vi "ProgG_011_MG.vi"() -> ()   [LabVIEW 2021]
panel:
  out "Wynik":ext=1.0
  in  "x":ext
  in  "?":bool
  # "Oblicz wartoœæ  sinc(x)"
  # "Oblicz wartoœæ sin(x)"
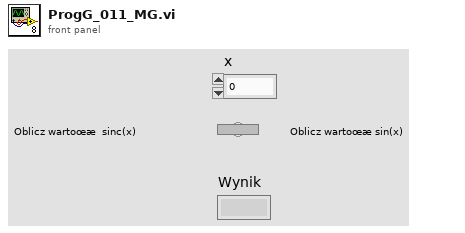
[diagram p1: front panel]
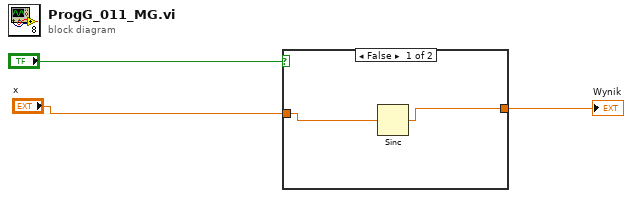
[diagram p0: block diagram]
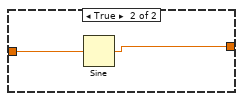
[diagram p2: hidden frame]
diagram:
  n1 = case shown="False" "?" {
    tunnel: "x" -> [w5 w7]
    tunnel: [w4 w6] -> w1
    frame False {
      n2 = Sinc(1:w5) -> (0:w4:ext)
    }
    frame True {
      n3 = Sine(x=w7) -> (sin(x)=w6:ext)
    }
  }
  "Wynik" <- w1
